vi "RMSData.vi"(9 "Data in":dbl[](array[numeric]), 10 "t":dbl, 11 "Fs":dbl) -> (3 "RMS Data out":dbl[](array[numeric]))   [LabVIEW 2019]
uses:
  <vilib>/Analysis/5stat.llb/RMS (DBL).vi
  <vilib>/Analysis/NI_AALPro.lvlib
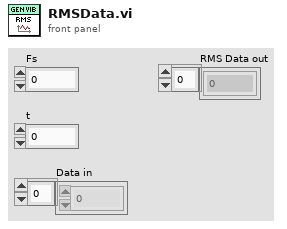
[diagram p1: front panel]
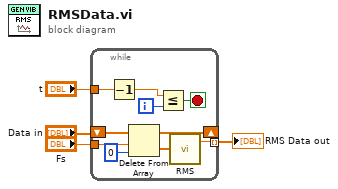
[diagram p0: block diagram]
diagram:
  n1 = while {
    tunnel: "Fs" -> [w12]
    shift-right: [w11] -> _
    shift-left: "Data in" -> [w14]
    tunnel: [w5] -> w4 mode=indexing
    tunnel: "t" -> [w8]
    i -> [w10]
    stop <- w9 stop-if-true
    n2 = Decrement(x=w8) -> (x-1=w7:dbl)
    n3 = Delete From Array(array=w14, length=w12, index=0) -> (deleted portion=w6:dbl[], array with subset deleted=w11:dbl[])
    n4 = Less Or Equal?(x=w7, y=w10) -> (x <= y?=w9:bool)
    n5 = call-poly <vilib>:"RMS.vi"("X"=w6) -> ("rms value"=w5:dbl)  [unwired: 1 out]
  }
  "RMS Data out" <- w4
